vi "Apply Texture (no reference).vi"(4 "Blend Color":T1, 5 "Vertical Wrap Mode":enum16{"Clamp", "Repeat"}(ring), 6 "Filter Mode":T2(ring), 7 "Horizontal Wrap Mode":enum16{"Clamp", "Repeat"}(ring), 8 "error in (no error)":errorcluster, 9 "Apply Mode":T4(ring), 10 "Image Data":T3, 11 "Scene Object In":refnum<vi>) -> (0 "error out":errorcluster, 3 "Scene Object Out":refnum<vi>)   [LabVIEW 2020, in "NI_3D Picture Control.lvlib"]
doc: "Maps a texture to the surface of a 3D object. You must manually select the polymorphic instance to use."
uses:
  <vilib>/picture/3D Picture Control/NI_3D Picture Control.lvlib
  <vilib>/picture/picture.llb/imagedata.ctl
  <vilib>/Utility/miscctls.llb/LVRGBAColorTypeDef.ctl
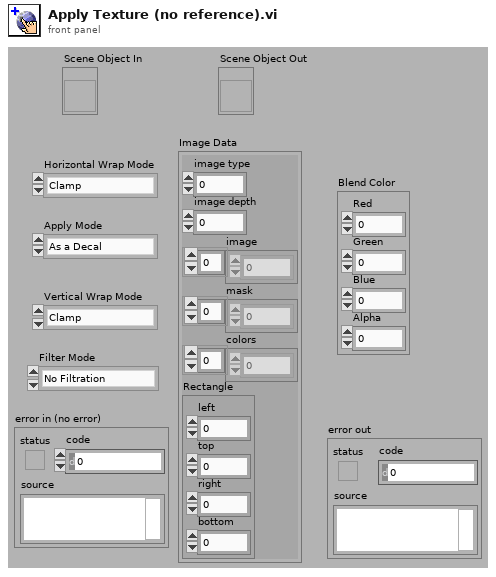
[diagram p1: front panel]
types:
  T1 = typedef "LVRGBAColorTypeDef.ctl" = cluster{"Red":sgl, "Green":sgl, "Blue":sgl, "Alpha":sgl}
  T2 = enum16{"No Filtration", "Linear Filtration", "Simple Mipmap Filtration", "Bilinear Filtration", "Trilinear Filtration"}
  T3 = typedef "imagedata.ctl" = cluster{"image type":i32, "image depth":i32, "image":u8[], "mask":u8[], "colors":u32[], "Rectangle":cluster{"left":i16, "top":i16, "right":i16, "bottom":i16}}
  T4 = enum16{"As a Decal", "With Modulation", "With Blending", "As a replacement"}
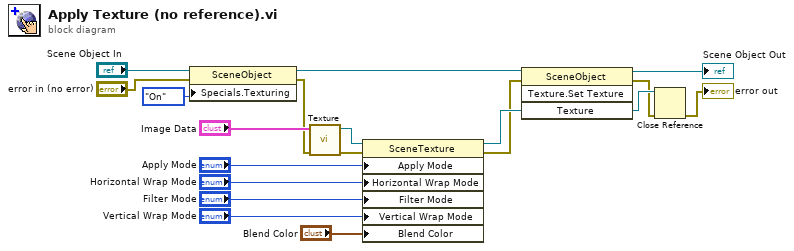
[diagram p0: block diagram]
diagram:
  n1 = property class="SceneObject"(reference="Scene Object In", error in="error in (no error)", "Specials.Texturing"=enum16{"Inherit Value", "Off", "On"}."On" ("Specials:Texturing")) -> (reference out=w13:refnum<vi>, error out=w8:errorcluster)
  n2 = call <vilib>:"Texture.vi"("error in (no error)"=w8, "Image"="Image Data") -> ("error out"=w10:errorcluster, "New Texture Refnum"=w15:refnum<vi>)  [unwired: 8 out]
  n3 = property class="SceneTexture"(reference=w15, error in=w10, "Apply Mode"="Apply Mode", "Horizontal Wrap Mode"="Horizontal Wrap Mode", "Filter Mode"="Filter Mode", "Vertical Wrap Mode"="Vertical Wrap Mode", "Blend Color"="Blend Color") -> (reference out=w17:refnum<vi>, error out=w7:errorcluster)
  n4 = invoke class="SceneObject" method="Texture.Set Texture"(reference=w13, error in=w7, "Texture"=w17) -> (reference out=→"Scene Object Out":refnum<vi>, error out=w2:errorcluster, "Texture"=w3:refnum<vi>)  [unwired: 1 in, 1 out]
  n5 = Close Reference(reference=w3, error in (no error)=w2) -> (error out=→"error out":errorcluster)
